vi "Eval Condition.vi"(7 "Variables":refnum<class "Variables.lvclass">, 8 "error in (no error)":errorcluster, 9 "Sequence Time":T1, 11 "Time Condition in":refnum<class "Time Condition.lvclass">) -> (0 "error out":errorcluster, 2 "Result":bool, 3 "Time Condition out":refnum<class "Time Condition.lvclass">)   [LabVIEW 2020, in "VolatusSeq.lvlib" / "Time Condition.lvclass"]
uses:
  Time Condition.lvclass
  Sequence Time.ctl
  Variables/Variables.lvclass
  Time Condition.lvclass/Time Condition.ctl
  VolatusSeq.lvlib
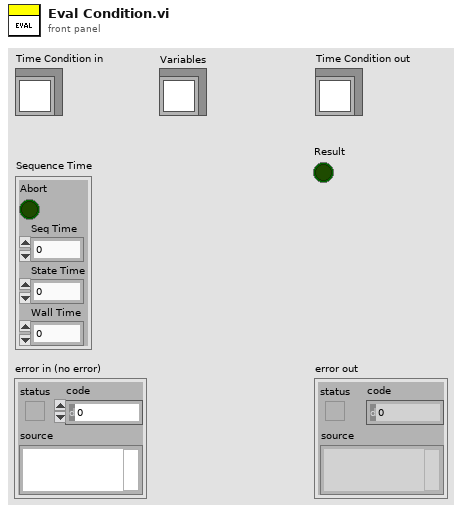
[diagram p1: front panel]
types:
  T1 = typedef "VolatusSeq.lvlib/Sequence Time.ctl" = cluster{"Abort":bool, "Seq Time":dbl, "State Time":dbl, "Wall Time":dbl}
  T2 = typedef "VolatusSeqConfig.lvlib/Timer.ctl" = enum16{"Sequence", "State", "Wall"}
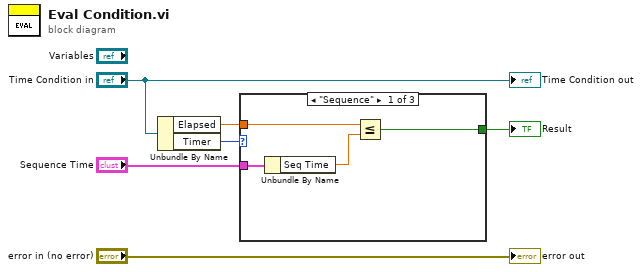
[diagram p0: block diagram]
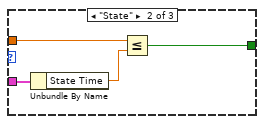
[diagram p2: hidden frame]
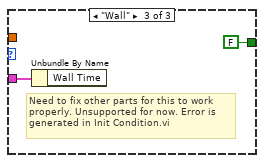
[diagram p3: hidden frame]
diagram:
  n1 = Unbundle By Name("Time Condition in") -> ("Elapsed"=w3:dbl, "Timer"=w4:T2)
  n2 = case shown="\"Sequence\"" w4 {
    tunnel: w3 -> [w7 w13 _]
    tunnel: "Sequence Time" -> [w10 w14 w16]
    tunnel: [w9 w11 FALSE] -> w1
    frame "Sequence" {
      n3 = Unbundle By Name(w10) -> ("Seq Time"=w8:dbl)
      n4 = Less Or Equal?(x=w7, y=w8) -> (x <= y?=w9:bool)
    }
    frame "State" {
      n5 = Unbundle By Name(w14) -> ("State Time"=w12:dbl)
      n6 = Less Or Equal?(x=w13, y=w12) -> (x <= y?=w11:bool)
    }
    frame "Wall" {
      # "Need to fix other parts for this to work properly. Unsupported for now. Error is generated in Init Condition.vi"
      n7 = Unbundle By Name(w16) -> ()  [unwired: 1 out]
    }
  }
  "Result" <- w1
  "error out" <- "error in (no error)"
  "Time Condition out" <- "Time Condition in"
